vi "Uninit.vi"(2 "Container State":T1, 3 "Display State":T2) -> ()   [LabVIEW 2017, in "XY Plot Matrix.xctl"]
uses:
  <vilib>/Math Plots/2D Math Plots/XY Plot Matrix/XY Plot Matrix XCtrl/XY Plot Matrix.xctl
  <vilib>/Math Plots/2D Math Plots/XY Plot Matrix/XY Plot Matrix XCtrl/State.ctl
  <vilib>/Math Plots/2D Math Plots/XY Plot Matrix/XY Plot Matrix/XY Plot Matrix.lvclass
  <vilib>/Math Plots/2D Math Plots/2D Plot/Action String/XYPlotMatrix Ctrl Act Queue.ctl
  <vilib>/Math Plots/2D Math Plots/2D Plot/Action String/XYPlotMatrix Ctrl Act Cluster.ctl
  <vilib>/Math Plots/2D Math Plots/2D Plot/Action String/2DMathPlot State Class.ctl
  <vilib>/_xctls/Container State.ctl
  <vilib>/_xctls/XControlSupport.lvlib
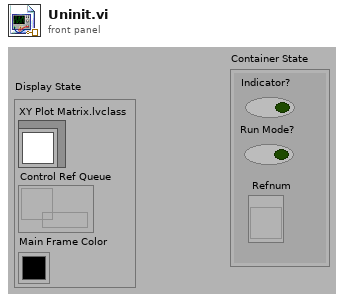
[diagram p1: front panel]
types:
  T1 = typedef "XControlSupport.lvlib/Container State.ctl" = cluster{"Indicator?":bool, "Run Mode?":bool, " Refnum":refnum<vi>}
  T2 = typedef "XY Plot Matrix.xctl/State.ctl" = cluster{"XY Plot Matrix.lvclass":refnum<class "XY Plot Matrix.lvclass">, "Control Ref Queue":T3, "Main Frame Color":u32}
  T3 = typedef "XYPlotMatrix Ctrl Act Queue.ctl" = refnum<queue>
  T4 = typedef "XYPlotMatrix Ctrl Act Cluster.ctl" = cluster{"Facade VI":refnum<vi>, "XControl":refnum<vi>, "Sub Panel":refnum<vi>, "Sub VI":refnum<vi>, "Export Image":refnum<vi>, "Display State Change Class":T5}
  T5 = typedef "2DMathPlot State Class.ctl" = enum16{"Update All (Undo)", "Update General", "Update Appearance", "Update Format", "Update Scale", "Update Marker", "Update Cursor", "None"}
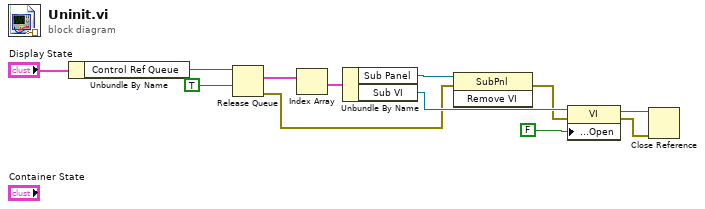
[diagram p0: block diagram]
diagram:
  n1 = Unbundle By Name("Display State") -> ("Control Ref Queue"=w11:T3)
  n2 = Release Queue(queue=w11, force destroy? (F)=TRUE) -> (remaining elements=w9:T4[], error out=w1:errorcluster)  [unwired: 1 in, 1 out]
  n3 = Index Array(array=w9) -> (element=w8:T4)  [unwired: 1 in]
  n4 = Unbundle By Name(w8) -> ("Sub Panel"=w3:refnum<vi>, "Sub VI"=w7:refnum<vi>)
  n5 = invoke class="SubPnl" method="Remove VI"(reference=w3, error in=w1) -> (error out=w2:errorcluster)  [unwired: 1 in, 2 out]
  n6 = property class="VI"(reference=w7, error in=w2, "Front Panel.Open"=FALSE ("Front Panel Window:Open")) -> (reference out=w5:refnum<vi>, error out=w4:errorcluster)
  n7 = Close Reference(reference=w5, error in (no error)=w4) -> ()  [unwired: 1 out]
